vi "Test Config Update.vi"(0 "StringRefArray":refnum<vi>[](array[refnum]), 2 "Mode":enum16{"Init", "Clear", "Update"}(ring)=enum."Clear", 7 "Pump Control Style":refnum<vi>, 11 "TestCfgCluster":T2) -> (4 "Pump Control Style Out":T1)   [LabVIEW 2013]
uses:
  TypeDef/Controller Names.ctl
  TypeDef/TestCfgCluster.ctl
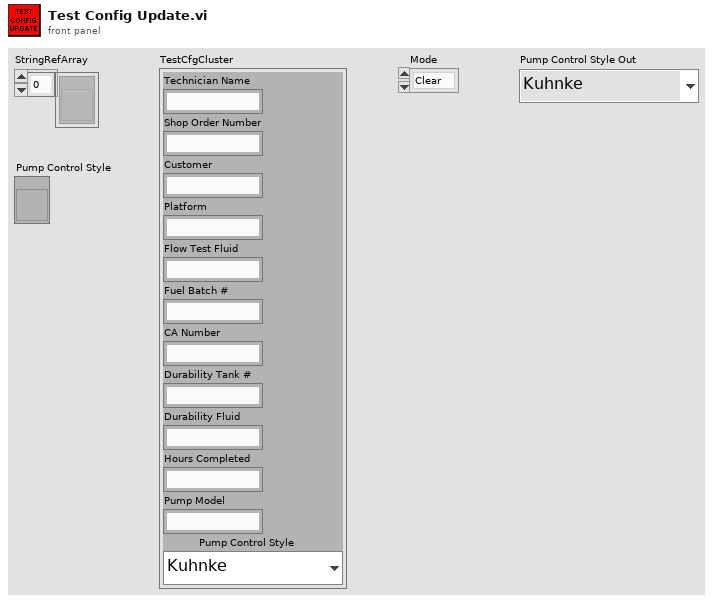
[diagram p1: front panel]
types:
  T1 = typedef "Controller Names.ctl" = enum16{"Kuhnke", "McLaren", "Helbako BLDC", "Conti", "Hella E4LMF", "Hella E4LMD", "Hella E4DCG 20mm", "Hella E4DCG 30mm", "Helbako (old)", "TI PWM", "PSA", "Hella Hyundai Gas", "Hella Hyundai Diesel", "8 Comm", "10 Comm", "8 Comm Hella FCA", "10 Comm Hella FCA", "8 Comm Omron", "10 Comm Omron", "8 Comm Nissan", "10 Comm Nissan"}
  T2 = typedef "TestCfgCluster.ctl" = cluster{"Technician Name":string, "Shop Order Number":string, "Customer":string, "Platform":string, "Flow Test Fluid":string, "Fuel Batch #":string, "CA Number":string, "Durability Tank #":string, "Durability Fluid":string, "Hours Completed":string, "Pump Model":string, "Pump Control Style":T1}
  T3 = cluster{"CA Number":string, "Shop Order Number":string, "Customer":string, "Platform":string, "Flow Test Fluid":string, "Fuel Batch #":string, "Pump Model":string, "Technician Name":string, "Durability Tank #":string, "Durability Fluid":string, "Hours Completed":string}
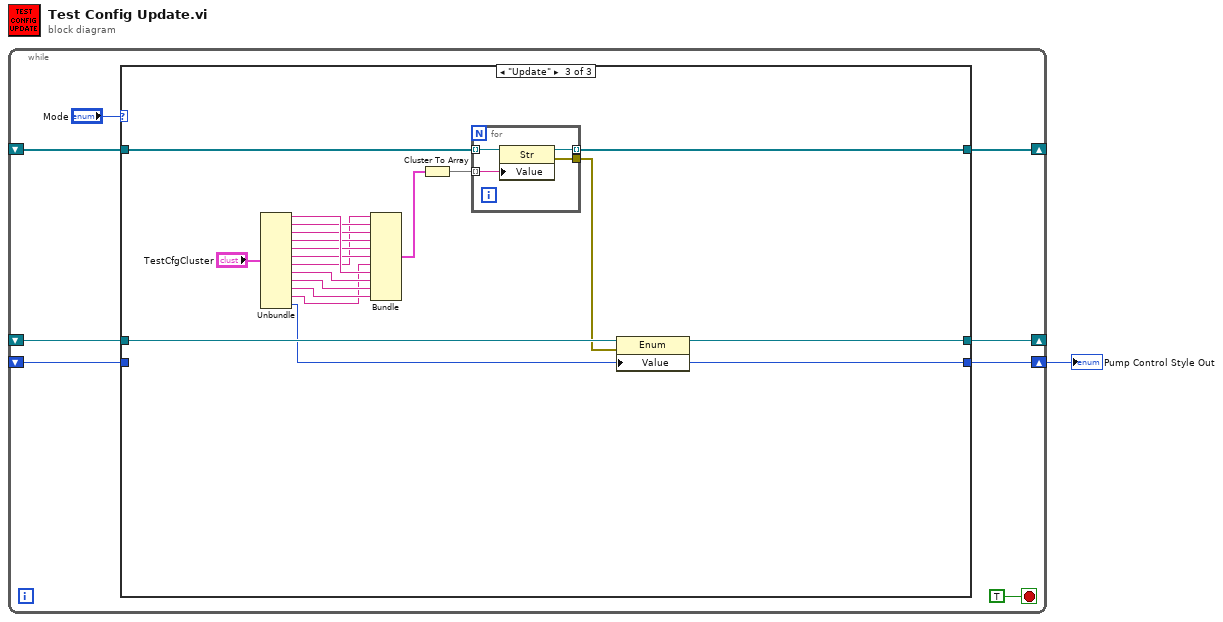
[diagram p0: block diagram]
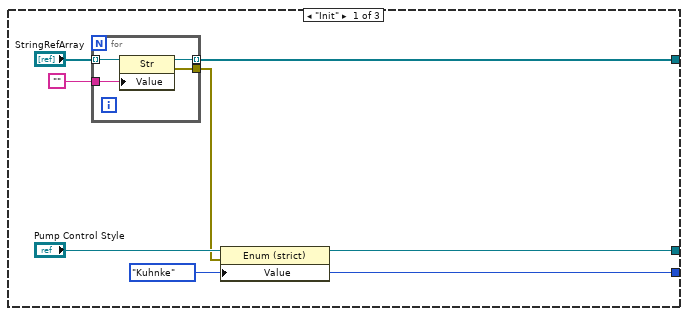
[diagram p2: hidden frame]
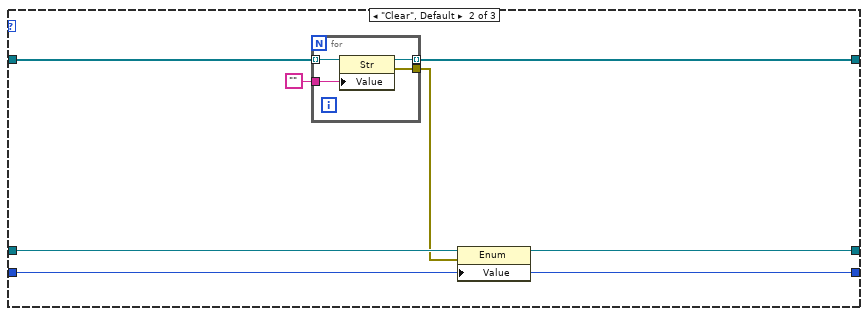
[diagram p3: hidden frame]
diagram:
  n1 = while {
    shift-right: [w7] -> _
    shift-left: _ -> [w6]
    shift-right: [w5] -> _
    shift-left: _ -> [w3]
    shift-right: [w4] -> w1
    shift-left: _ -> [w2]
    stop <- TRUE stop-if-true
    n2 = case shown="\"Update\"" "Mode" {
      tunnel: [w15 w26 w50] -> w7
      tunnel: w6 -> [_ w27 w51]
      tunnel: [w11 w23 w47] -> w5
      tunnel: [w10 w24 w43] -> w4
      tunnel: w3 -> [_ w25 w49]
      tunnel: w2 -> [_ w24 _]
      frame "Init" {
        w10 = Controller_Names."Kuhnke" ("Value")
        n3 = for {
          tunnel: "StringRefArray" -> [w20] mode=indexing
          tunnel: [w19] -> w12
          tunnel: [w18] -> w15 mode=indexing
          tunnel: "" -> [w17]
          n4 = property on="Property Node" class="Str"(reference=w20, "Value"=w17) -> (reference out=w18:refnum<vi>, error out=w19:errorcluster)  [unwired: 1 in]
        }
        n5 = property on="Property Node" class="Enum (strict)"(reference="Pump Control Style", error in=w12, "Value"=w10) -> (reference out=w11:refnum<vi>)  [unwired: 1 out]
      }
      frame "Clear", Default {
        n6 = for {
          tunnel: w27 -> [w31] mode=indexing
          tunnel: [w30] -> w22
          tunnel: [w29] -> w26 mode=indexing
          tunnel: "" -> [w28]
          n7 = property on="Property Node" class="Str"(reference=w31, "Value"=w28) -> (reference out=w29:refnum<vi>, error out=w30:errorcluster)  [unwired: 1 in]
        }
        n8 = property on="Property Node" class="Enum"(reference=w25, error in=w22, "Value"=w24) -> (reference out=w23:refnum<vi>)  [unwired: 1 out]
      }
      frame "Update" {
        n9 = Unbundle("TestCfgCluster") -> ("Technician Name"=w42:string, "Shop Order Number"=w41:string, "Customer"=w40:string, "Platform"=w39:string, "Flow Test Fluid"=w38:string, "Fuel Batch #"=w37:string, "CA Number"=w36:string, "Durability Tank #"=w35:string, "Durability Fluid"=w34:string, "Hours Completed"=w33:string, "Pump Model"=w32:string, "Pump Control Style"=w43:T1)
        n10 = Bundle("CA Number"=w36, "Shop Order Number"=w41, "Customer"=w40, "Platform"=w39, "Flow Test Fluid"=w38, "Fuel Batch #"=w37, "Pump Model"=w32, "Technician Name"=w42, "Durability Tank #"=w35, "Durability Fluid"=w34, "Hours Completed"=w33) -> (w45:T3)  [unwired: 1 in]
        n11 = Cluster To Array(cluster=w45) -> (array=w44:string[])
        n12 = for {
          tunnel: w51 -> [w55] mode=indexing
          tunnel: [w54] -> w48
          tunnel: [w53] -> w50 mode=indexing
          tunnel: w44 -> [w52] mode=indexing
          n13 = property on="Property Node" class="Str"(reference=w55, "Value"=w52) -> (reference out=w53:refnum<vi>, error out=w54:errorcluster)  [unwired: 1 in]
        }
        n14 = property on="Property Node" class="Enum"(reference=w49, error in=w48, "Value"=w43) -> (reference out=w47:refnum<vi>)  [unwired: 1 out]
      }
    }
  }
  "Pump Control Style Out" <- w1
